vi "Repartidor_coloresB.vi"() -> ()   [LabVIEW 2017]
uses:
  <extravilib>/ChannelInstances/Stream-bool/Read With Abort.vi
  <extravilib>/ChannelInstances/Stream-bool/Write With Abort.vi
  <extravilib>/ChannelInstances/Stream-bool/EndpointRead.vi
  <extravilib>/ChannelInstances/Stream-bool/Endpoint.vi
  <extravilib>/ChannelInstances/Stream-bool/Instantiate.vi
  <extravilib>/ChannelInstances/Stream-bool/)Channel.vi
  <resource>/ChannelSupport/_ChannelSupport/WaitIfNeeded.vi
  <extravilib>/ChannelInstances/Stream-bool.lvlib
panel:
  in  "Consumidor":u32=100
  in  "Productor":u32=100
  out "A 10":u32[][](array[colorbox])
  out "A 9":u32[][](array[colorbox])
  out "A 8":u32[][](array[colorbox])
  out "A 7":u32[][](array[colorbox])
  out "A 6":u32[][](array[colorbox])
  out "A 5":u32[][](array[colorbox])
  out "A 4":u32[][](array[colorbox])
  out "A 3":u32[][](array[colorbox])
  out "A 2":u32[][](array[colorbox])
  out "A":u32[][](array[colorbox])
  in  "stop":bool
  out "Color Box":u32(colorbox)
  out "Array 2":u32[](array[colorbox])
  out "Array":u32[][](array[colorbox])
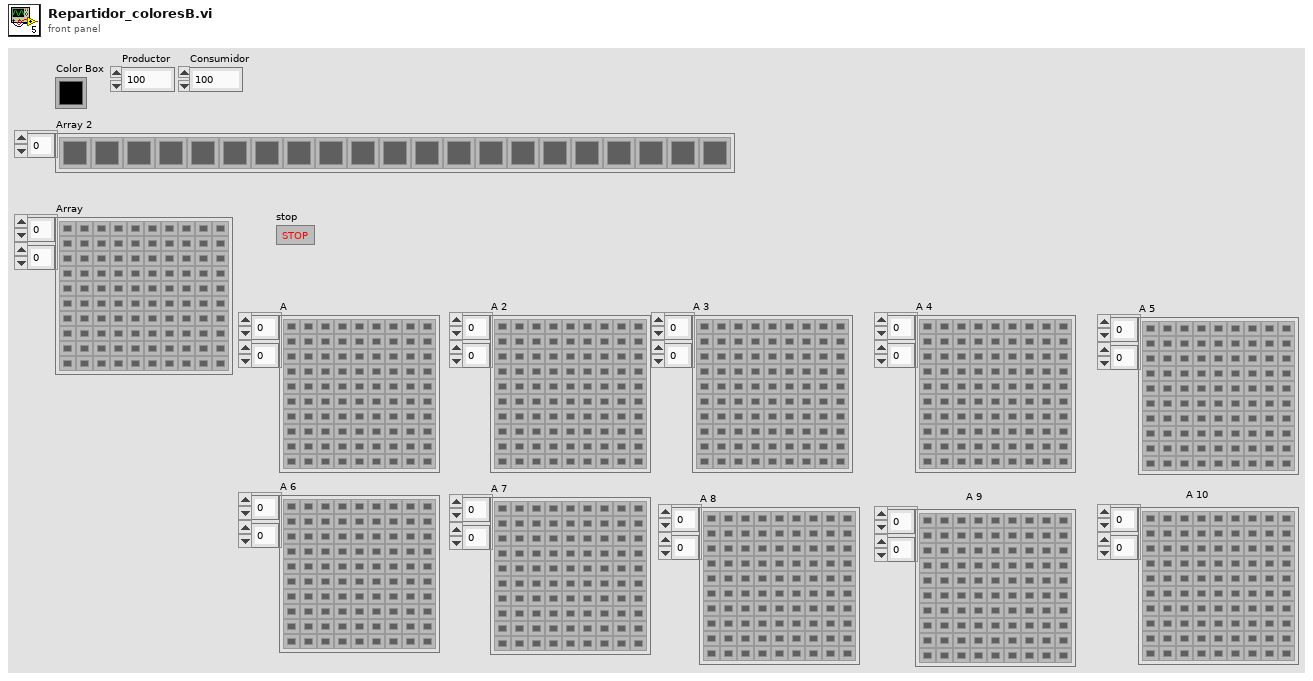
[diagram p1: front panel]
types:
  T1 = cluster{"Numeros":u32[], "A1":u32[], "B1":u32[], "C1":u32[], "D1":u32[], "E1":u32[], "F1":u32[], "G1":u32[], "H1":u32[], "I1":u32[], "J1":u32[]}
  T2 = typedef "Stream-bool.lvlib/)Channel.ctl" = refnum<queue>
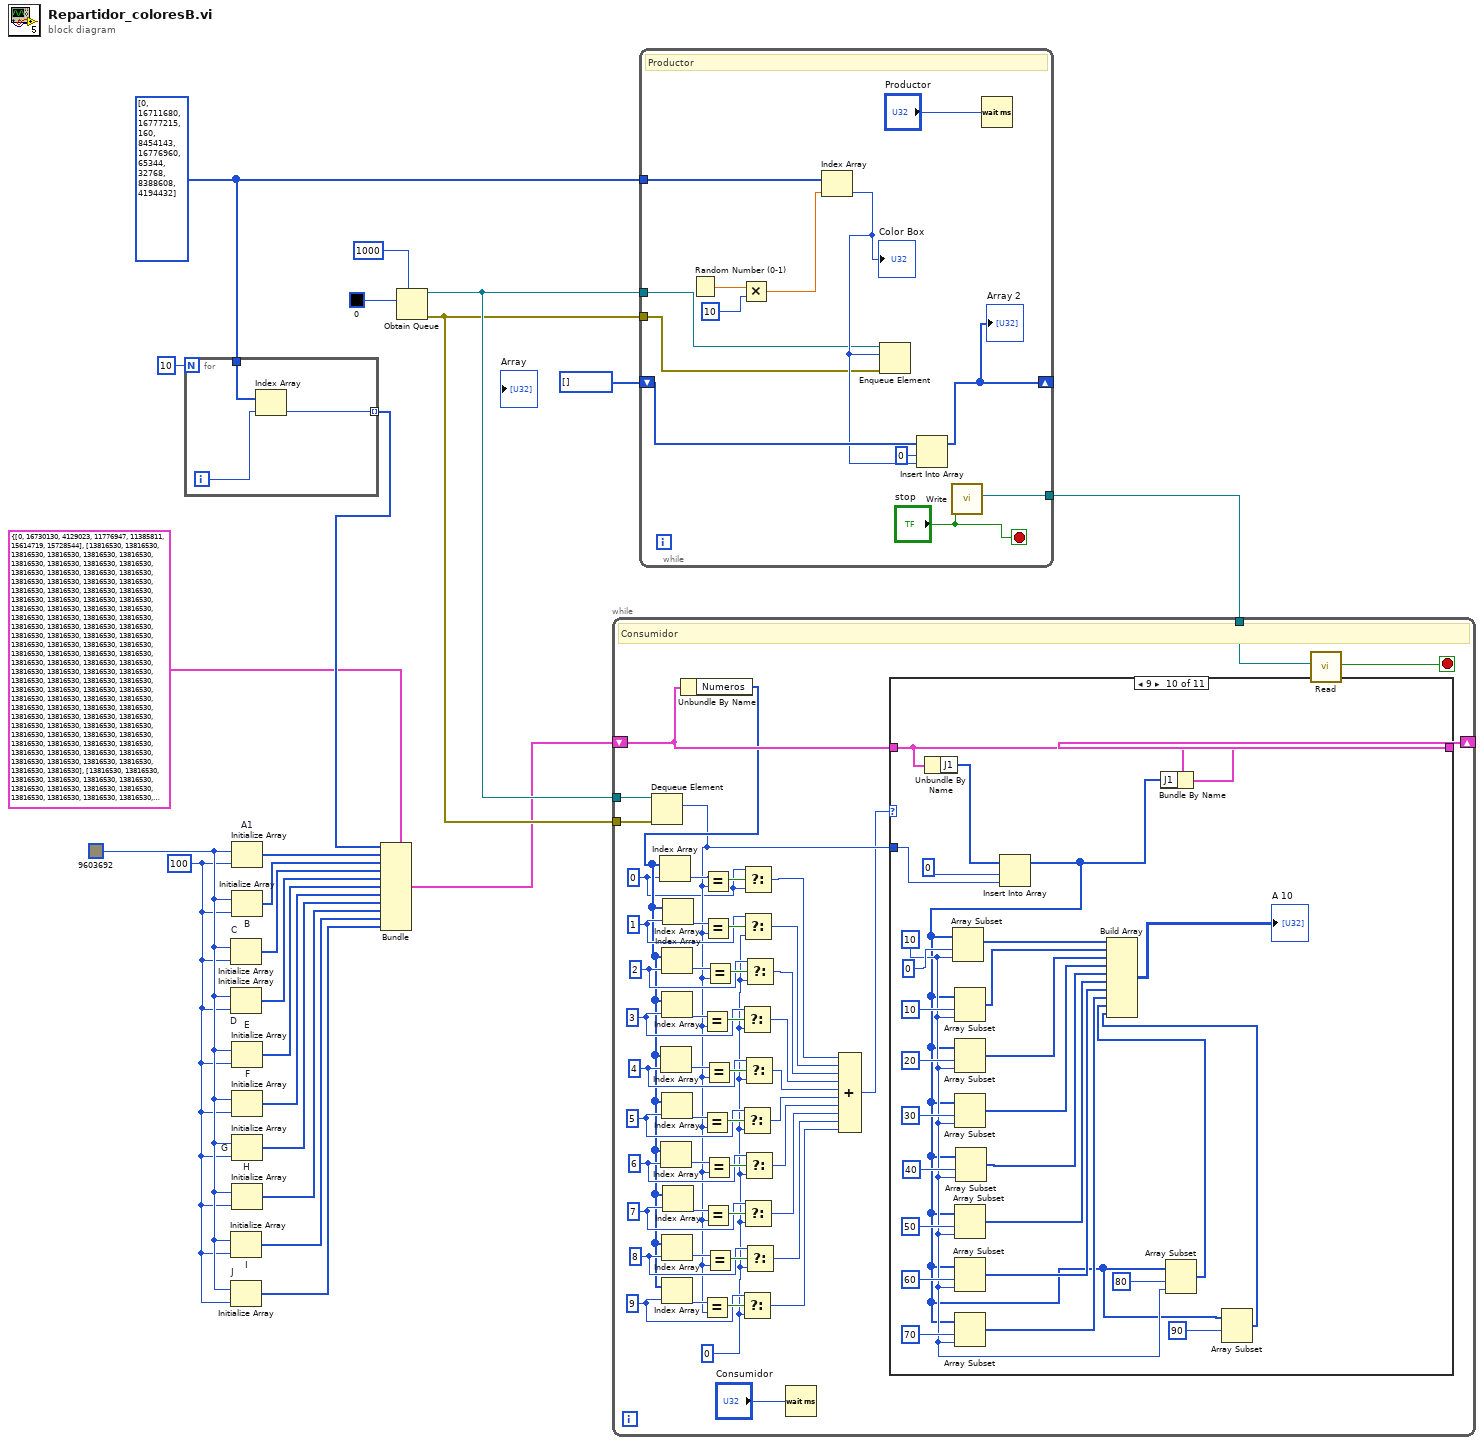
[diagram p0: block diagram]
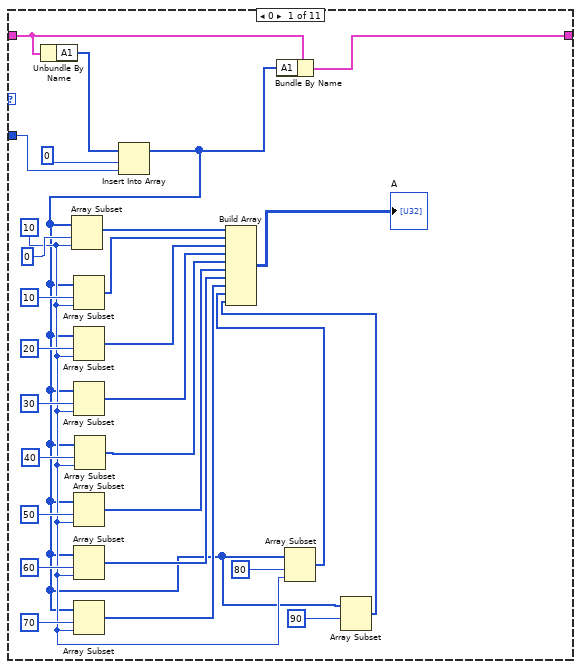
[diagram p2: hidden frame]
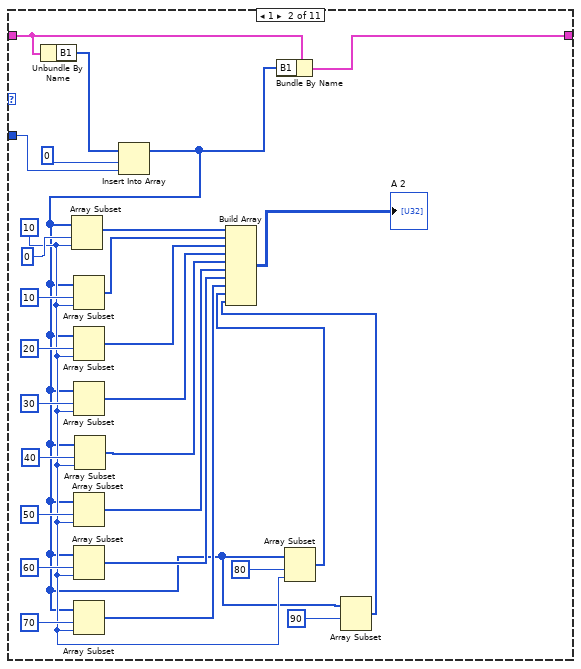
[diagram p3: hidden frame]
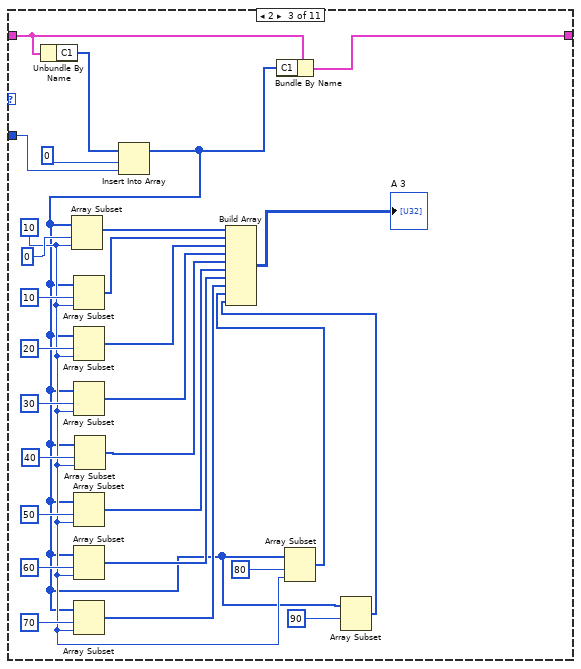
[diagram p4: hidden frame]
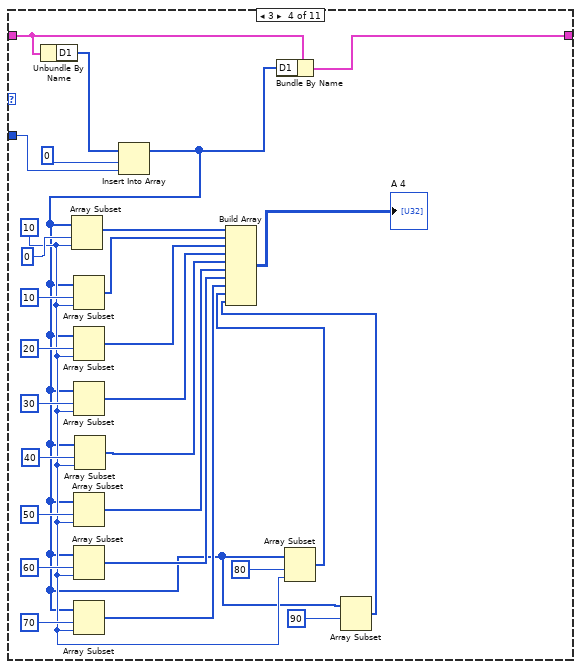
[diagram p5: hidden frame]
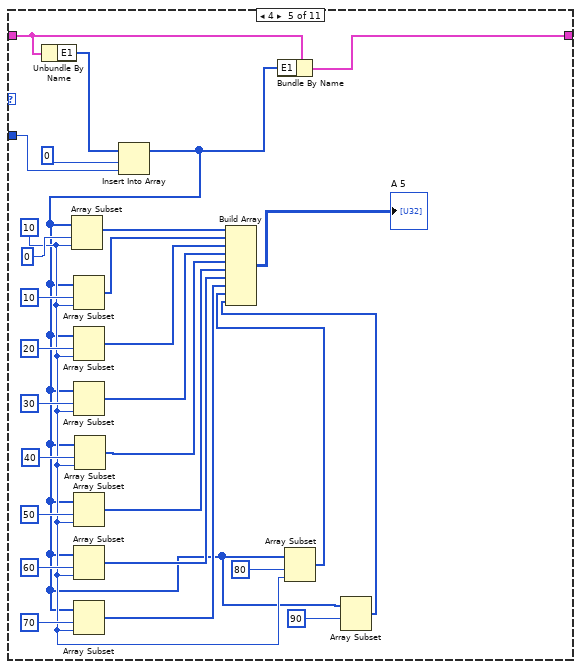
[diagram p6: hidden frame]
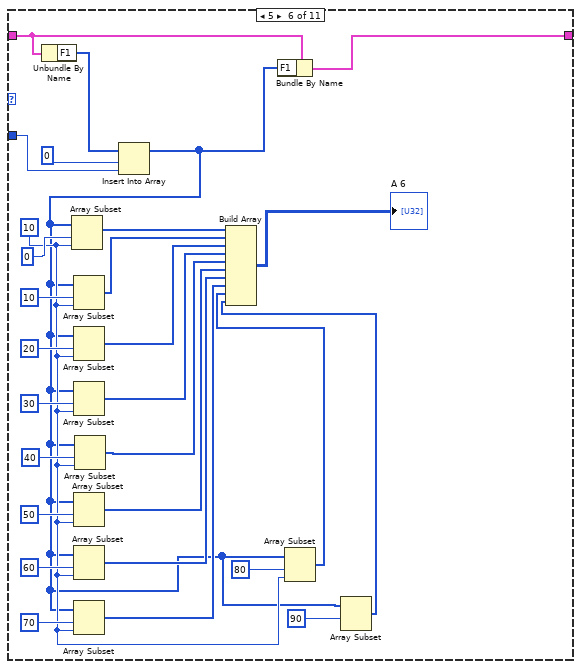
[diagram p7: hidden frame]
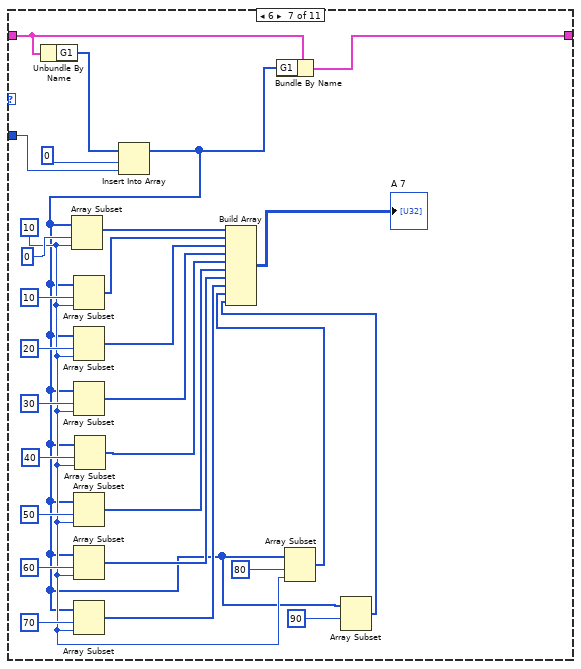
[diagram p8: hidden frame]
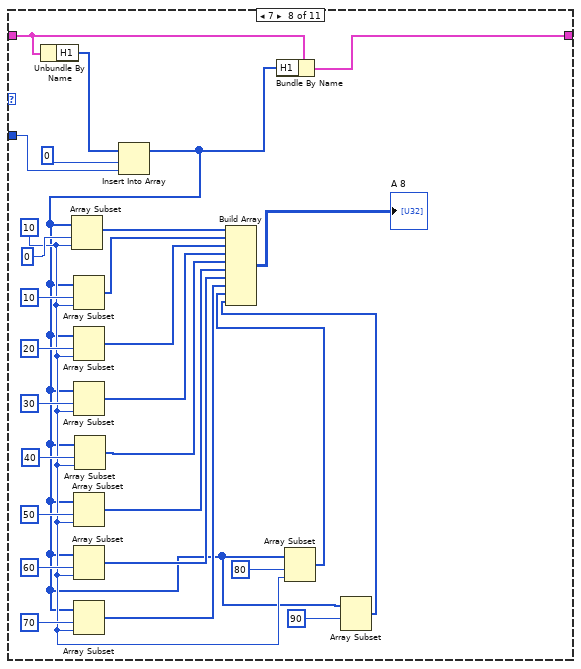
[diagram p9: hidden frame]
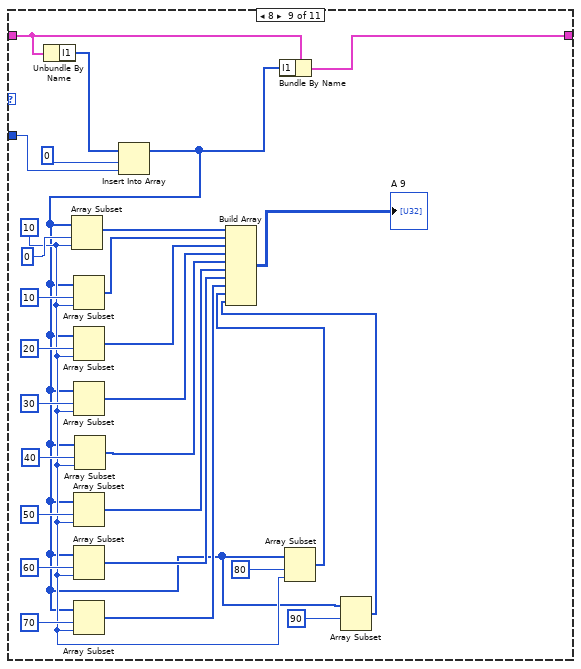
[diagram p10: hidden frame]
diagram:
  w3 = u32[] [0, 16711680, 16777215, 160, 8454143, 16776960, 65344, 32768, 8388608, 4194432]
  w18 = u32 9603692
  w17 = 100 ("dimension size")
  n1 = for {
    N: 10 -> [_]
    tunnel: w3 -> [w26]
    tunnel: [w24] -> w8 mode=indexing
    i -> [w25]
    n2 = Index Array "Index Array"(array=w26, index=w25) -> (element=w24:u32)
  }
  n3 = Initialize Array "C"(w18, w17) -> (w16:u32[])
  n4 = Initialize Array "D"(w18, w17) -> (w15:u32[])
  n5 = Initialize Array "I"(w18, w17) -> (w10:u32[])
  n6 = Initialize Array "J"(w18, w17) -> (w1:u32[])
  n7 = Initialize Array "A1"(w18, w17) -> (w6:u32[])
  n8 = Initialize Array "B"(w18, w17) -> (w7:u32[])
  n9 = Initialize Array "E"(w18, w17) -> (w14:u32[])
  n10 = Initialize Array "F"(w18, w17) -> (w13:u32[])
  n11 = Initialize Array "G"(w18, w17) -> (w12:u32[])
  n12 = Initialize Array "H"(w18, w17) -> (w11:u32[])
  n13 = Bundle "Bundle"(cluster=T1 {"Numeros"=[0, 16730130, 4129023, 11776947, 11385811, 15614719, 15728544], "A1"=[13816530, 13816530, 13816530, 13816530, 13816530, 13816530, 13816530, 13816530, 13816530, 13816530, 13816530, 13816530, 13816530, 13816530, 13816530, 13816530, 13816530, 13816530, 13816530, 13816530, 13816530, 13816530, 13816530, 13816530, 13816530, 13816530, 13816530, 13816530, 13816530, 13816530, 13816530, 13816530, 13816530, 13816530, 13816530, 13816530, 13816530, 13816530, 13816530, 13816530, 13816530, 13816530, 13816530, 13816530, 13816530, 13816530, 13816530, 13816530, 13816530, 13816530, 13816530, 13816530, 13816530, 13816530, 13816530, 13816530, 13816530, 13816530, 13816530, 13816530, 13816530, 13816530, 13816530, 13816530, 13816530, 13816530, 13816530, 13816530, 13816530, 13816530, 13816530, 13816530, 13816530, 13816530, 13816530, 13816530, 13816530, 13816530, 13816530, 13816530, 13816530, 13816530, 13816530, 13816530, 13816530, 13816530, 13816530, 13816530, 13816530, 13816530, 13816530, 13816530, 13816530, 13816530, 13816530, 13816530, 13816530, 13816530, 13816530, 13816530], "B1"=[13816530, 13816530, 13816530, 13816530, 13816530, 13816530, 13816530, 13816530, 13816530, 13816530, 13816530, 13816530, 13816530, 13816530, 13816530, 13816530, 13816530, 13816530, 13816530, 13816530, 13816530, 13816530, 13816530, 13816530, 13816530, 13816530, 13816530, 13816530, 13816530, 13816530, 13816530, 13816530, 13816530, 13816530, 13816530, 13816530, 13816530, 13816530, 13816530, 13816530, 13816530, 13816530, 13816530, 13816530, 13816530, 13816530, 13816530, 13816530, 13816530, 13816530, 13816530, 13816530, 13816530, 13816530, 13816530, 13816530, 13816530, 13816530, 13816530, 13816530, 13816530, 13816530, 13816530, 13816530, 13816530, 13816530, 13816530, 13816530, 13816530, 13816530, 13816530, 13816530, 13816530, 13816530, 13816530, 13816530, 13816530, 13816530, 13816530, 13816530, 13816530, 13816530, 13816530, 13816530, 13816530, 13816530, 13816530, 13816530, 13816530, 13816530, 13816530, 13816530, 13816530, 13816530, 13816530, 13816530, 13816530, 13816530, 13816530, 13816530], "C1"=[13816530, 13816530, 13816530, 13816530, 13816530, 13816530, 13816530, 13816530, 13816530, 13816530, 13816530, 13816530, 13816530, 13816530, 13816530, 13816530, 13816530, 13816530, 13816530, 13816530, 13816530, 13816530, 13816530, 13816530, 13816530, 13816530, 13816530, 13816530, 13816530, 13816530, 13816530, 13816530, 13816530, 13816530, 13816530, 13816530, 13816530, 13816530, 13816530, 13816530, 13816530, 13816530, 13816530, 13816530, 13816530, 13816530, 13816530, 13816530, 13816530, 13816530, 13816530, 13816530, 13816530, 13816530, 13816530, 13816530, 13816530, 13816530, 13816530, 13816530, 13816530, 13816530, 13816530, 13816530, 13816530, 13816530, 13816530, 13816530, 13816530, 13816530, 13816530, 13816530, 13816530, 13816530, 13816530, 13816530, 13816530, 13816530, 13816530, 13816530, 13816530, 13816530, 13816530, 13816530, 13816530, 13816530, 13816530, 13816530, 13816530, 13816530, 13816530, 13816530, 13816530, 13816530, 13816530, 13816530, 13816530, 13816530, 13816530, 13816530], "D1"=[13816530, 13816530, 13816530, 13816530, 13816530, 13816530, 13816530, 13816530, 13816530, 13816530, 13816530, 13816530, 13816530, 13816530, 13816530, 13816530, 13816530, 13816530, 13816530, 13816530, 13816530, 13816530, 13816530, 13816530, 13816530, 13816530, 13816530, 13816530, 13816530, 13816530, 13816530, 13816530, 13816530, 13816530, 13816530, 13816530, 13816530, 13816530, 13816530, 13816530, 13816530, 13816530, 13816530, 13816530, 13816530, 13816530, 13816530, 13816530, 13816530, 13816530, 13816530, 13816530, 13816530, 13816530, 13816530, 13816530, 13816530, 13816530, 13816530, 13816530, 13816530, 13816530, 13816530, 13816530, 13816530, 13816530, 13816530, 13816530, 13816530, 13816530, 13816530, 13816530, 13816530, 13816530, 13816530, 13816530, 13816530, 13816530, 13816530, 13816530, 13816530, 13816530, 13816530, 13816530, 13816530, 13816530, 13816530, 13816530, 13816530, 13816530, 13816530, 13816530, 13816530, 13816530, 13816530, 13816530, 13816530, 13816530, 13816530, 13816530], "E1"=[13816530, 13816530, 13816530, 13816530, 13816530, 13816530, 13816530, 13816530, 13816530, 13816530, 13816530, 13816530, 13816530, 13816530, 13816530, 13816530, 13816530, 13816530, 13816530, 13816530, 13816530, 13816530, 13816530, 13816530, 13816530, 13816530, 13816530, 13816530, 13816530, 13816530, 13816530, 13816530, 13816530, 13816530, 13816530, 13816530, 13816530, 13816530, 13816530, 13816530, 13816530, 13816530, 13816530, 13816530, 13816530, 13816530, 13816530, 13816530, 13816530, 13816530, 13816530, 13816530, 13816530, 13816530, 13816530, 13816530, 13816530, 13816530, 13816530, 13816530, 13816530, 13816530, 13816530, 13816530, 13816530, 13816530, 13816530, 13816530, 13816530, 13816530, 13816530, 13816530, 13816530, 13816530, 13816530, 13816530, 13816530, 13816530, 13816530, 13816530, 13816530, 13816530, 13816530, 13816530, 13816530, 13816530, 13816530, 13816530, 13816530, 13816530, 13816530, 13816530, 13816530, 13816530, 13816530, 13816530, 13816530, 13816530, 13816530, 13816530], "F1"=[13816530, 13816530, 13816530, 13816530, 13816530, 13816530, 13816530, 13816530, 13816530, 13816530, 13816530, 13816530, 13816530, 13816530, 13816530, 13816530, 13816530, 13816530, 13816530, 13816530, 13816530, 13816530, 13816530, 13816530, 13816530, 13816530, 13816530, 13816530, 13816530, 13816530, 13816530, 13816530, 13816530, 13816530, 13816530, 13816530, 13816530, 13816530, 13816530, 13816530, 13816530, 13816530, 13816530, 13816530, 13816530, 13816530, 13816530, 13816530, 13816530, 13816530, 13816530, 13816530, 13816530, 13816530, 13816530, 13816530, 13816530, 13816530, 13816530, 13816530, 13816530, 13816530, 13816530, 13816530, 13816530, 13816530, 13816530, 13816530, 13816530, 13816530, 13816530, 13816530, 13816530, 13816530, 13816530, 13816530, 13816530, 13816530, 13816530, 13816530, 13816530, 13816530, 13816530, 13816530, 13816530, 13816530, 13816530, 13816530, 13816530, 13816530, 13816530, 13816530, 13816530, 13816530, 13816530, 13816530, 13816530, 13816530, 13816530, 13816530], "G1"=[13816530, 13816530, 13816530, 13816530, 13816530, 13816530, 13816530, 13816530, 13816530, 13816530, 13816530, 13816530, 13816530, 13816530, 13816530, 13816530, 13816530, 13816530, 13816530, 13816530, 13816530, 13816530, 13816530, 13816530, 13816530, 13816530, 13816530, 13816530, 13816530, 13816530, 13816530, 13816530, 13816530, 13816530, 13816530, 13816530, 13816530, 13816530, 13816530, 13816530, 13816530, 13816530, 13816530, 13816530, 13816530, 13816530, 13816530, 13816530, 13816530, 13816530, 13816530, 13816530, 13816530, 13816530, 13816530, 13816530, 13816530, 13816530, 13816530, 13816530, 13816530, 13816530, 13816530, 13816530, 13816530, 13816530, 13816530, 13816530, 13816530, 13816530, 13816530, 13816530, 13816530, 13816530, 13816530, 13816530, 13816530, 13816530, 13816530, 13816530, 13816530, 13816530, 13816530, 13816530, 13816530, 13816530, 13816530, 13816530, 13816530, 13816530, 13816530, 13816530, 13816530, 13816530, 13816530, 13816530, 13816530, 13816530, 13816530, 13816530], "H1"=[13816530, 13816530, 13816530, 13816530, 13816530, 13816530, 13816530, 13816530, 13816530, 13816530, 13816530, 13816530, 13816530, 13816530, 13816530, 13816530, 13816530, 13816530, 13816530, 13816530, 13816530, 13816530, 13816530, 13816530, 13816530, 13816530, 13816530, 13816530, 13816530, 13816530, 13816530, 13816530, 13816530, 13816530, 13816530, 13816530, 13816530, 13816530, 13816530, 13816530, 13816530, 13816530, 13816530, 13816530, 13816530, 13816530, 13816530, 13816530, 13816530, 13816530, 13816530, 13816530, 13816530, 13816530, 13816530, 13816530, 13816530, 13816530, 13816530, 13816530, 13816530, 13816530, 13816530, 13816530, 13816530, 13816530, 13816530, 13816530, 13816530, 13816530, 13816530, 13816530, 13816530, 13816530, 13816530, 13816530, 13816530, 13816530, 13816530, 13816530, 13816530, 13816530, 13816530, 13816530, 13816530, 13816530, 13816530, 13816530, 13816530, 13816530, 13816530, 13816530, 13816530, 13816530, 13816530, 13816530, 13816530, 13816530, 13816530, 13816530], "I1"=[13816530, 13816530, 13816530, 13816530, 13816530, 13816530, 13816530, 13816530, 13816530, 13816530, 13816530, 13816530, 13816530, 13816530, 13816530, 13816530, 13816530, 13816530, 13816530, 13816530, 13816530, 13816530, 13816530, 13816530, 13816530, 13816530, 13816530, 13816530, 13816530, 13816530, 13816530, 13816530, 13816530, 13816530, 13816530, 13816530, 13816530, 13816530, 13816530, 13816530, 13816530, 13816530, 13816530, 13816530, 13816530, 13816530, 13816530, 13816530, 13816530, 13816530, 13816530, 13816530, 13816530, 13816530, 13816530, 13816530, 13816530, 13816530, 13816530, 13816530, 13816530, 13816530, 13816530, 13816530, 13816530, 13816530, 13816530, 13816530, 13816530, 13816530, 13816530, 13816530, 13816530, 13816530, 13816530, 13816530, 13816530, 13816530, 13816530, 13816530, 13816530, 13816530, 13816530, 13816530, 13816530, 13816530, 13816530, 13816530, 13816530, 13816530, 13816530, 13816530, 13816530, 13816530, 13816530, 13816530, 13816530, 13816530, 13816530, 13816530], "J1"=[13816530, 13816530, 13816530, 13816530, 13816530, 13816530, 13816530, 13816530, 13816530, 13816530, 13816530, 13816530, 13816530, 13816530, 13816530, 13816530, 13816530, 13816530, 13816530, 13816530, 13816530, 13816530, 13816530, 13816530, 13816530, 13816530, 13816530, 13816530, 13816530, 13816530, 13816530, 13816530, 13816530, 13816530, 13816530, 13816530, 13816530, 13816530, 13816530, 13816530, 13816530, 13816530, 13816530, 13816530, 13816530, 13816530, 13816530, 13816530, 13816530, 13816530, 13816530, 13816530, 13816530, 13816530, 13816530, 13816530, 13816530, 13816530, 13816530, 13816530, 13816530, 13816530, 13816530, 13816530, 13816530, 13816530, 13816530, 13816530, 13816530, 13816530, 13816530, 13816530, 13816530, 13816530, 13816530, 13816530, 13816530, 13816530, 13816530, 13816530, 13816530, 13816530, 13816530, 13816530, 13816530, 13816530, 13816530, 13816530, 13816530, 13816530, 13816530, 13816530, 13816530, 13816530, 13816530, 13816530, 13816530, 13816530, 13816530, 13816530]}, "Numeros"=w8, "A1"=w6, "B1"=w7, "C1"=w16, "D1"=w15, "E1"=w14, "F1"=w13, "G1"=w12, "H1"=w11, "I1"=w10, "J1"=w1) -> (w5:T1)
  n14 = Obtain Queue(max queue size (-1, unlimited)=1000, element data type=u32 0) -> (queue out=w20:refnum<queue>, error out=w19:errorcluster)  [unwired: 3 in, 1 out]
  n15 = while {
    shift-right: [w32] -> _
    shift-left: u32[] [] -> [w34]
    tunnel: w19 -> [w30]
    tunnel: w20 -> [w29]
    tunnel: w3 -> [w28]
    tunnel: [w27] -> w2
    stop <- "stop" stop-if-true
    # "Productor"
    n16 = Random Number (0-1)() -> (number: 0 to 1=w39:dbl)
    n17 = Multiply(x=w39, y=10) -> (x*y=w37:dbl)
    n18 = Index Array "Index Array"(array=w28, index=w37) -> (element=w31:u32)
    "Color Box" <- w31
    n19 = Enqueue Element(queue=w29, element=w31, error in (no error)=w30) -> ()  [unwired: 1 in, 3 out]
    n20 = Insert Into Array "Insert Into Array"(array=w34, index=0, new element=w31) -> (w32:u32[])
    "Array 2" <- w32
    n21 = call <extravilib>:"Write.vi"("element"="stop") -> ("channel"=w27:T2)  [unwired: 8 in, 2 out]
    n22 = Wait (ms)(milliseconds to wait="Productor") -> ()  [unwired: 1 out]
  }
  n23 = while {
    tunnel: w20 -> [w90]
    tunnel: w19 -> [w89]
    shift-right: [w88] -> _
    shift-left: w5 -> [w87]
    tunnel: w2 -> [w42]
    stop <- w41 stop-if-true
    w44 = 0 ("f")
    w67 = 9 ("index")
    w69 = 8 ("index")
    w71 = 7 ("index")
    w73 = 6 ("index")
    w75 = 5 ("index")
    w77 = 4 ("index")
    w79 = 3 ("index")
    w81 = 2 ("index")
    w83 = 1 ("index")
    w55 = 0 ("index")
    # "Consumidor"
    n24 = Dequeue Element(queue=w90, error in (no error)=w89) -> (element=w56:u32)  [unwired: 1 in, 3 out]
    n25 = Unbundle By Name(w87) -> ("Numeros"=w66:u32[])
    n26 = Index Array(array=w66, index=w55) -> (element=w86:u32)
    n27 = Index Array(array=w66, index=w77) -> (element=w60:u32)
    n28 = Index Array(array=w66, index=w73) -> (element=w62:u32)
    n29 = Index Array(array=w66, index=w81) -> (element=w58:u32)
    n30 = Index Array(array=w66, index=w79) -> (element=w59:u32)
    n31 = Index Array(array=w66, index=w75) -> (element=w61:u32)
    n32 = Index Array(array=w66, index=w69) -> (element=w64:u32)
    n33 = Index Array(array=w66, index=w67) -> (element=w65:u32)
    n34 = Index Array(array=w66, index=w83) -> (element=w57:u32)
    n35 = Index Array(array=w66, index=w71) -> (element=w63:u32)
    n36 = Equal?(x=w59, y=w56) -> (x = y?=w80:bool)
    n37 = Equal?(x=w61, y=w56) -> (x = y?=w76:bool)
    n38 = Equal?(x=w65, y=w56) -> (x = y?=w68:bool)
    n39 = Equal?(x=w86, y=w56) -> (x = y?=w85:bool)
    n40 = Equal?(x=w57, y=w56) -> (x = y?=w84:bool)
    n41 = Equal?(x=w63, y=w56) -> (x = y?=w72:bool)
    n42 = Equal?(x=w60, y=w56) -> (x = y?=w78:bool)
    n43 = Equal?(x=w62, y=w56) -> (x = y?=w74:bool)
    n44 = Equal?(x=w58, y=w56) -> (x = y?=w82:bool)
    n45 = Equal?(x=w64, y=w56) -> (x = y?=w70:bool)
    n46 = Select(t=w79, s=w80, f=w44) -> (s? t:f=w51:i32)
    n47 = Select(t=w75, s=w76, f=w44) -> (s? t:f=w49:i32)
    n48 = Select(t=w67, s=w68, f=w44) -> (s? t:f=w45:i32)
    n49 = Select(t=w55, s=w85, f=w55) -> (s? t:f=w54:i32)
    n50 = Select(t=w83, s=w84, f=w44) -> (s? t:f=w53:i32)
    n51 = Select(t=w71, s=w72, f=w44) -> (s? t:f=w47:i32)
    n52 = Select(t=w77, s=w78, f=w44) -> (s? t:f=w50:i32)
    n53 = Select(t=w73, s=w74, f=w44) -> (s? t:f=w48:i32)
    n54 = Select(t=w81, s=w82, f=w44) -> (s? t:f=w52:i32)
    n55 = Select(t=w69, s=w70, f=w44) -> (s? t:f=w46:i32)
    n56 = Wait (ms)(milliseconds to wait="Consumidor") -> ()  [unwired: 1 out]
    n57 = Compound Arithmetic op=ADD(w54, w53, w52, w51, w50, w49, w48, w47, w46, w45) -> (w43:i32)
    n58 = case shown="9" w43 {
      tunnel: w87 -> [w114 w142 w170 w198 w226 w254 w282 w310 w338 w366 w371]
      tunnel: [w116 w144 w172 w200 w228 w256 w284 w312 w340 w368 w371] -> w88
      tunnel: w56 -> [w115 w143 w171 w199 w227 w255 w283 w311 w339 w367 _]
      frame 0 {
        w101 = 10 ("length")
        n59 = Unbundle By Name(w114) -> ("A1"=w117:u32[])
        n60 = Insert Into Array "Insert Into Array"(array=w117, index=0, new element=w115) -> (w92:u32[])
        n61 = Array Subset "Array Subset"(array=w92, index=0 ("length"), length=w101) -> (w113:u32[])
        n62 = Array Subset "Array Subset"(array=w92, index=10, length=w101) -> (w111:u32[])
        n63 = Array Subset "Array Subset"(array=w92, index=20, length=w101) -> (w100:u32[])
        n64 = Array Subset "Array Subset"(array=w92, index=30, length=w101) -> (w99:u32[])
        n65 = Array Subset "Array Subset"(array=w92, index=50, length=w101) -> (w97:u32[])
        n66 = Array Subset "Array Subset"(array=w92, index=60, length=w101) -> (w96:u32[])
        n67 = Array Subset "Array Subset"(array=w92, index=70, length=w101) -> (w95:u32[])
        n68 = Array Subset "Array Subset"(array=w92, index=40, length=w101) -> (w98:u32[])
        n69 = Bundle By Name(cluster=w114, "A1"=w92) -> (w116:T1)
        n70 = Array Subset "Array Subset"(array=w92, index=80, length=w101) -> (w94:u32[])
        n71 = Array Subset "Array Subset"(array=w92, index=90) -> (w91:u32[])  [unwired: 1 in]
        n72 = Build Array(w113, w111, w100, w99, w98, w97, w96, w95, w94, w91) -> (→"A":u32[][])
      }
      frame 1 {
        w129 = 10 ("length")
        n73 = Unbundle By Name(w142) -> ("B1"=w145:u32[])
        n74 = Insert Into Array "Insert Into Array"(array=w145, index=0, new element=w143) -> (w120:u32[])
        n75 = Array Subset "Array Subset"(array=w120, index=0 ("length"), length=w129) -> (w141:u32[])
        n76 = Array Subset "Array Subset"(array=w120, index=10, length=w129) -> (w139:u32[])
        n77 = Array Subset "Array Subset"(array=w120, index=20, length=w129) -> (w128:u32[])
        n78 = Array Subset "Array Subset"(array=w120, index=30, length=w129) -> (w127:u32[])
        n79 = Array Subset "Array Subset"(array=w120, index=50, length=w129) -> (w125:u32[])
        n80 = Array Subset "Array Subset"(array=w120, index=60, length=w129) -> (w124:u32[])
        n81 = Array Subset "Array Subset"(array=w120, index=70, length=w129) -> (w123:u32[])
        n82 = Array Subset "Array Subset"(array=w120, index=40, length=w129) -> (w126:u32[])
        n83 = Bundle By Name(cluster=w142, "B1"=w120) -> (w144:T1)
        n84 = Array Subset "Array Subset"(array=w120, index=80, length=w129) -> (w122:u32[])
        n85 = Array Subset "Array Subset"(array=w120, index=90) -> (w119:u32[])  [unwired: 1 in]
        n86 = Build Array(w141, w139, w128, w127, w126, w125, w124, w123, w122, w119) -> (→"A 2":u32[][])
      }
      frame 2 {
        w157 = 10 ("length")
        n87 = Unbundle By Name(w170) -> ("C1"=w173:u32[])
        n88 = Insert Into Array "Insert Into Array"(array=w173, index=0, new element=w171) -> (w148:u32[])
        n89 = Array Subset "Array Subset"(array=w148, index=0 ("length"), length=w157) -> (w169:u32[])
        n90 = Array Subset "Array Subset"(array=w148, index=10, length=w157) -> (w167:u32[])
        n91 = Array Subset "Array Subset"(array=w148, index=20, length=w157) -> (w156:u32[])
        n92 = Array Subset "Array Subset"(array=w148, index=30, length=w157) -> (w155:u32[])
        n93 = Array Subset "Array Subset"(array=w148, index=50, length=w157) -> (w153:u32[])
        n94 = Array Subset "Array Subset"(array=w148, index=60, length=w157) -> (w152:u32[])
        n95 = Array Subset "Array Subset"(array=w148, index=70, length=w157) -> (w151:u32[])
        n96 = Array Subset "Array Subset"(array=w148, index=40, length=w157) -> (w154:u32[])
        n97 = Bundle By Name(cluster=w170, "C1"=w148) -> (w172:T1)
        n98 = Array Subset "Array Subset"(array=w148, index=80, length=w157) -> (w150:u32[])
        n99 = Array Subset "Array Subset"(array=w148, index=90) -> (w147:u32[])  [unwired: 1 in]
        n100 = Build Array(w169, w167, w156, w155, w154, w153, w152, w151, w150, w147) -> (→"A 3":u32[][])
      }
      frame 3 {
        w185 = 10 ("length")
        n101 = Unbundle By Name(w198) -> ("D1"=w201:u32[])
        n102 = Insert Into Array "Insert Into Array"(array=w201, index=0, new element=w199) -> (w176:u32[])
        n103 = Array Subset "Array Subset"(array=w176, index=0 ("length"), length=w185) -> (w197:u32[])
        n104 = Array Subset "Array Subset"(array=w176, index=10, length=w185) -> (w195:u32[])
        n105 = Array Subset "Array Subset"(array=w176, index=20, length=w185) -> (w184:u32[])
        n106 = Array Subset "Array Subset"(array=w176, index=30, length=w185) -> (w183:u32[])
        n107 = Array Subset "Array Subset"(array=w176, index=50, length=w185) -> (w181:u32[])
        n108 = Array Subset "Array Subset"(array=w176, index=60, length=w185) -> (w180:u32[])
        n109 = Array Subset "Array Subset"(array=w176, index=70, length=w185) -> (w179:u32[])
        n110 = Array Subset "Array Subset"(array=w176, index=40, length=w185) -> (w182:u32[])
        n111 = Bundle By Name(cluster=w198, "D1"=w176) -> (w200:T1)
        n112 = Array Subset "Array Subset"(array=w176, index=80, length=w185) -> (w178:u32[])
        n113 = Array Subset "Array Subset"(array=w176, index=90) -> (w175:u32[])  [unwired: 1 in]
        n114 = Build Array(w197, w195, w184, w183, w182, w181, w180, w179, w178, w175) -> (→"A 4":u32[][])
      }
      frame 4 {
        w213 = 10 ("length")
        n115 = Unbundle By Name(w226) -> ("E1"=w229:u32[])
        n116 = Insert Into Array "Insert Into Array"(array=w229, index=0, new element=w227) -> (w204:u32[])
        n117 = Array Subset "Array Subset"(array=w204, index=0 ("length"), length=w213) -> (w225:u32[])
        n118 = Array Subset "Array Subset"(array=w204, index=10, length=w213) -> (w223:u32[])
        n119 = Array Subset "Array Subset"(array=w204, index=20, length=w213) -> (w212:u32[])
        n120 = Array Subset "Array Subset"(array=w204, index=30, length=w213) -> (w211:u32[])
        n121 = Array Subset "Array Subset"(array=w204, index=50, length=w213) -> (w209:u32[])
        n122 = Array Subset "Array Subset"(array=w204, index=60, length=w213) -> (w208:u32[])
        n123 = Array Subset "Array Subset"(array=w204, index=70, length=w213) -> (w207:u32[])
        n124 = Array Subset "Array Subset"(array=w204, index=40, length=w213) -> (w210:u32[])
        n125 = Bundle By Name(cluster=w226, "E1"=w204) -> (w228:T1)
        n126 = Array Subset "Array Subset"(array=w204, index=80, length=w213) -> (w206:u32[])
        n127 = Array Subset "Array Subset"(array=w204, index=90) -> (w203:u32[])  [unwired: 1 in]
        n128 = Build Array(w225, w223, w212, w211, w210, w209, w208, w207, w206, w203) -> (→"A 5":u32[][])
      }
      frame 5 {
        w241 = 10 ("length")
        n129 = Unbundle By Name(w254) -> ("F1"=w257:u32[])
        n130 = Insert Into Array "Insert Into Array"(array=w257, index=0, new element=w255) -> (w232:u32[])
        n131 = Array Subset "Array Subset"(array=w232, index=0 ("length"), length=w241) -> (w253:u32[])
        n132 = Array Subset "Array Subset"(array=w232, index=10, length=w241) -> (w251:u32[])
        n133 = Array Subset "Array Subset"(array=w232, index=20, length=w241) -> (w240:u32[])
        n134 = Array Subset "Array Subset"(array=w232, index=30, length=w241) -> (w239:u32[])
        n135 = Array Subset "Array Subset"(array=w232, index=50, length=w241) -> (w237:u32[])
        n136 = Array Subset "Array Subset"(array=w232, index=60, length=w241) -> (w236:u32[])
        n137 = Array Subset "Array Subset"(array=w232, index=70, length=w241) -> (w235:u32[])
        n138 = Array Subset "Array Subset"(array=w232, index=40, length=w241) -> (w238:u32[])
        n139 = Bundle By Name(cluster=w254, "F1"=w232) -> (w256:T1)
        n140 = Array Subset "Array Subset"(array=w232, index=80, length=w241) -> (w234:u32[])
        n141 = Array Subset "Array Subset"(array=w232, index=90) -> (w231:u32[])  [unwired: 1 in]
        n142 = Build Array(w253, w251, w240, w239, w238, w237, w236, w235, w234, w231) -> (→"A 6":u32[][])
      }
      frame 6 {
        w269 = 10 ("length")
        n143 = Unbundle By Name(w282) -> ("G1"=w285:u32[])
        n144 = Insert Into Array "Insert Into Array"(array=w285, index=0, new element=w283) -> (w260:u32[])
        n145 = Array Subset "Array Subset"(array=w260, index=0 ("length"), length=w269) -> (w281:u32[])
        n146 = Array Subset "Array Subset"(array=w260, index=10, length=w269) -> (w279:u32[])
        n147 = Array Subset "Array Subset"(array=w260, index=20, length=w269) -> (w268:u32[])
        n148 = Array Subset "Array Subset"(array=w260, index=30, length=w269) -> (w267:u32[])
        n149 = Array Subset "Array Subset"(array=w260, index=50, length=w269) -> (w265:u32[])
        n150 = Array Subset "Array Subset"(array=w260, index=60, length=w269) -> (w264:u32[])
        n151 = Array Subset "Array Subset"(array=w260, index=70, length=w269) -> (w263:u32[])
        n152 = Array Subset "Array Subset"(array=w260, index=40, length=w269) -> (w266:u32[])
        n153 = Bundle By Name(cluster=w282, "G1"=w260) -> (w284:T1)
        n154 = Array Subset "Array Subset"(array=w260, index=80, length=w269) -> (w262:u32[])
        n155 = Array Subset "Array Subset"(array=w260, index=90) -> (w259:u32[])  [unwired: 1 in]
        n156 = Build Array(w281, w279, w268, w267, w266, w265, w264, w263, w262, w259) -> (→"A 7":u32[][])
      }
      frame 7 {
        w297 = 10 ("length")
        n157 = Unbundle By Name(w310) -> ("H1"=w313:u32[])
        n158 = Insert Into Array "Insert Into Array"(array=w313, index=0, new element=w311) -> (w288:u32[])
        n159 = Array Subset "Array Subset"(array=w288, index=0 ("length"), length=w297) -> (w309:u32[])
        n160 = Array Subset "Array Subset"(array=w288, index=10, length=w297) -> (w307:u32[])
        n161 = Array Subset "Array Subset"(array=w288, index=20, length=w297) -> (w296:u32[])
        n162 = Array Subset "Array Subset"(array=w288, index=30, length=w297) -> (w295:u32[])
        n163 = Array Subset "Array Subset"(array=w288, index=50, length=w297) -> (w293:u32[])
        n164 = Array Subset "Array Subset"(array=w288, index=60, length=w297) -> (w292:u32[])
        n165 = Array Subset "Array Subset"(array=w288, index=70, length=w297) -> (w291:u32[])
        n166 = Array Subset "Array Subset"(array=w288, index=40, length=w297) -> (w294:u32[])
        n167 = Bundle By Name(cluster=w310, "H1"=w288) -> (w312:T1)
        n168 = Array Subset "Array Subset"(array=w288, index=80, length=w297) -> (w290:u32[])
        n169 = Array Subset "Array Subset"(array=w288, index=90) -> (w287:u32[])  [unwired: 1 in]
        n170 = Build Array(w309, w307, w296, w295, w294, w293, w292, w291, w290, w287) -> (→"A 8":u32[][])
      }
      frame 8 {
        w325 = 10 ("length")
        n171 = Unbundle By Name(w338) -> ("I1"=w341:u32[])
        n172 = Insert Into Array "Insert Into Array"(array=w341, index=0, new element=w339) -> (w316:u32[])
        n173 = Array Subset "Array Subset"(array=w316, index=0 ("length"), length=w325) -> (w337:u32[])
        n174 = Array Subset "Array Subset"(array=w316, index=10, length=w325) -> (w335:u32[])
        n175 = Array Subset "Array Subset"(array=w316, index=20, length=w325) -> (w324:u32[])
        n176 = Array Subset "Array Subset"(array=w316, index=30, length=w325) -> (w323:u32[])
        n177 = Array Subset "Array Subset"(array=w316, index=50, length=w325) -> (w321:u32[])
        n178 = Array Subset "Array Subset"(array=w316, index=60, length=w325) -> (w320:u32[])
        n179 = Array Subset "Array Subset"(array=w316, index=70, length=w325) -> (w319:u32[])
        n180 = Array Subset "Array Subset"(array=w316, index=40, length=w325) -> (w322:u32[])
        n181 = Bundle By Name(cluster=w338, "I1"=w316) -> (w340:T1)
        n182 = Array Subset "Array Subset"(array=w316, index=80, length=w325) -> (w318:u32[])
        n183 = Array Subset "Array Subset"(array=w316, index=90) -> (w315:u32[])  [unwired: 1 in]
        n184 = Build Array(w337, w335, w324, w323, w322, w321, w320, w319, w318, w315) -> (→"A 9":u32[][])
      }
      frame 9 {
        w353 = 10 ("length")
        n185 = Unbundle By Name(w366) -> ("J1"=w369:u32[])
        n186 = Insert Into Array "Insert Into Array"(array=w369, index=0, new element=w367) -> (w344:u32[])
        n187 = Array Subset "Array Subset"(array=w344, index=0 ("length"), length=w353) -> (w365:u32[])
        n188 = Array Subset "Array Subset"(array=w344, index=10, length=w353) -> (w363:u32[])
        n189 = Array Subset "Array Subset"(array=w344, index=20, length=w353) -> (w352:u32[])
        n190 = Array Subset "Array Subset"(array=w344, index=30, length=w353) -> (w351:u32[])
        n191 = Array Subset "Array Subset"(array=w344, index=50, length=w353) -> (w349:u32[])
        n192 = Array Subset "Array Subset"(array=w344, index=60, length=w353) -> (w348:u32[])
        n193 = Array Subset "Array Subset"(array=w344, index=70, length=w353) -> (w347:u32[])
        n194 = Array Subset "Array Subset"(array=w344, index=40, length=w353) -> (w350:u32[])
        n195 = Bundle By Name(cluster=w366, "J1"=w344) -> (w368:T1)
        n196 = Array Subset "Array Subset"(array=w344, index=80, length=w353) -> (w346:u32[])
        n197 = Array Subset "Array Subset"(array=w344, index=90) -> (w343:u32[])  [unwired: 1 in]
        n198 = Build Array(w365, w363, w352, w351, w350, w349, w348, w347, w346, w343) -> (→"A 10":u32[][])
      }
      frame 10, Default {
      }
    }
    n199 = call <extravilib>:"Read.vi"("channel"=w42) -> ("element"=w41:bool)  [unwired: 6 in, 4 out]
  }
